vi "CtrlTreeOpenApp.vi"(9 "AppPaths":map{string, string}(c390), 10 "AppName":string, 11 "TreeControl in":refnum<vi>) -> (3 "Application out":refnum<vi>)   [LabVIEW 2019]
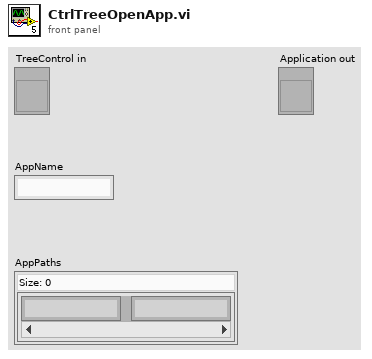
[diagram p1: front panel]
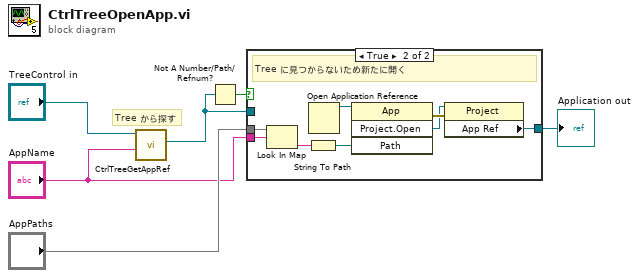
[diagram p0: block diagram]
diagram:
  # "Tree から探す"
  n1 = call "CtrlTreeGetAppRef.vi"("App Tag"="AppName", "ControlTree in"="TreeControl in") -> ("Application out"=w3:refnum<vi>)  [unwired: 6 in, 3 out]
  n2 = Not A Number/Path/Refnum?(number/path/refnum=w3) -> (NaN/Path/Refnum?=w2:bool)
  n3 = case shown="True" w2 {
    tunnel: w3 -> [w7 _]
    tunnel: [w7 w8] -> w4
    tunnel: "AppPaths" -> [_ w14]
    tunnel: "AppName" -> [_ w15]
    frame False {
    }
    frame True {
      # "Tree に見つからないため新たに開く"
      n4 = Look In Map(map=w14, key=w15) -> (value=w12:string)  [unwired: 1 in, 1 out]
      n5 = String To Path(string=w12) -> (path=w11:path)
      n6 = Open Application Reference() -> (3:w13:refnum<vi>)  [unwired: 4 in, 1 out]
      n7 = invoke class="App" method="Project.Open"(reference=w13, "Path"=w11) -> (error out=w10:errorcluster, "Project:Open"=w9:refnum<vi>)  [unwired: 2 in, 2 out]
      n8 = property class="Project"(reference=w9, error in=w10) -> ("App Ref"=w8:refnum<vi>)  [unwired: 2 out]
    }
  }
  "Application out" <- w4
